vi "niDTS WLAN UTIL chains array to chains.vi"(10 "Chains Array":bool[](array[boolean])=[TRUE, FALSE, FALSE, FALSE]) -> (2 "Chains":T1)   [LabVIEW 2015, in "niDTS WLAN.lvlib"]
uses:
  niDTS WLAN.lvlib
  Includes/niDTS WLAN INC Chains.ctl
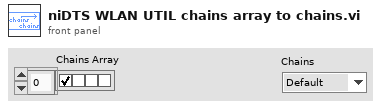
[diagram p1: front panel]
types:
  T1 = typedef "niDTS WLAN.lvlib/niDTS WLAN INC Chains.ctl" = enum16{"Default", "Chain 0", "Chain 1", "Chain 2", "Chain 3", "Chain 0 and 1", "Chain 2 and 3", "Chain 1,2 and 3", "Chains 1 - 4"}
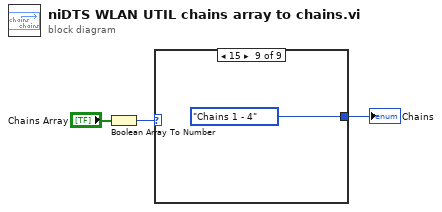
[diagram p0: block diagram]
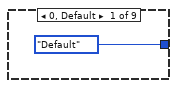
[diagram p2: hidden frame]
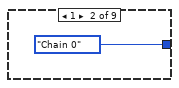
[diagram p3: hidden frame]
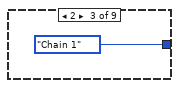
[diagram p4: hidden frame]
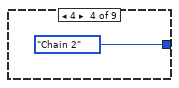
[diagram p5: hidden frame]
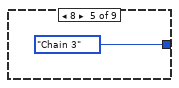
[diagram p6: hidden frame]
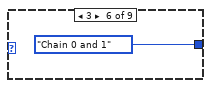
[diagram p7: hidden frame]
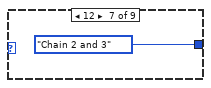
[diagram p8: hidden frame]
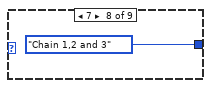
[diagram p9: hidden frame]
diagram:
  n1 = Boolean Array To Number(Boolean array="Chains Array") -> (number=w2:u32)
  n2 = case shown="15" w2 {
    tunnel: [niDTS_WLAN_INC_Chains."Default" ("Chains") niDTS_WLAN_INC_Chains."Chain 0" ("Chains") niDTS_WLAN_INC_Chains."Chain 1" ("Chains") niDTS_WLAN_INC_Chains."Chain 2" ("Chains") niDTS_WLAN_INC_Chains."Chain 3" ("Chains") niDTS_WLAN_INC_Chains."Chain 0 and 1" ("Chains") niDTS_WLAN_INC_Chains."Chain 2 and 3" ("Chains") niDTS_WLAN_INC_Chains."Chain 1,2 and 3" ("Chains") niDTS_WLAN_INC_Chains."Chains 1 - 4" ("Chains")] -> w1
    frame 0, Default {
    }
    frame 1 {
    }
    frame 2 {
    }
    frame 4 {
    }
    frame 8 {
    }
    frame 3 {
    }
    frame 12 {
    }
    frame 7 {
    }
    frame 15 {
    }
  }
  "Chains" <- w1
